vi "IVCV_measurement.vi"() -> ()   [LabVIEW 2016]
uses:
  <vilib>/Utility/file.llb/Read Delimited Spreadsheet (DBL).vi
panel:
  out "Channels":cluster{i32[], dbl[]}[](graph) caption="XY Graph"
  in  "Switch Delay (s)":dbl format="%#_13g"
  out "Voltages":cluster{"X":dbl[], "Y":dbl[]}[](graph) caption="XY Graph"
  in  "Voltage Delay (s)":dbl format="%#_13g"
  out "Input file":path
  in  "Sensor type":enum16{"6''", "8''"}(ring)
  in  "Measurement type":enum16{"IV", "CV"}(ring)
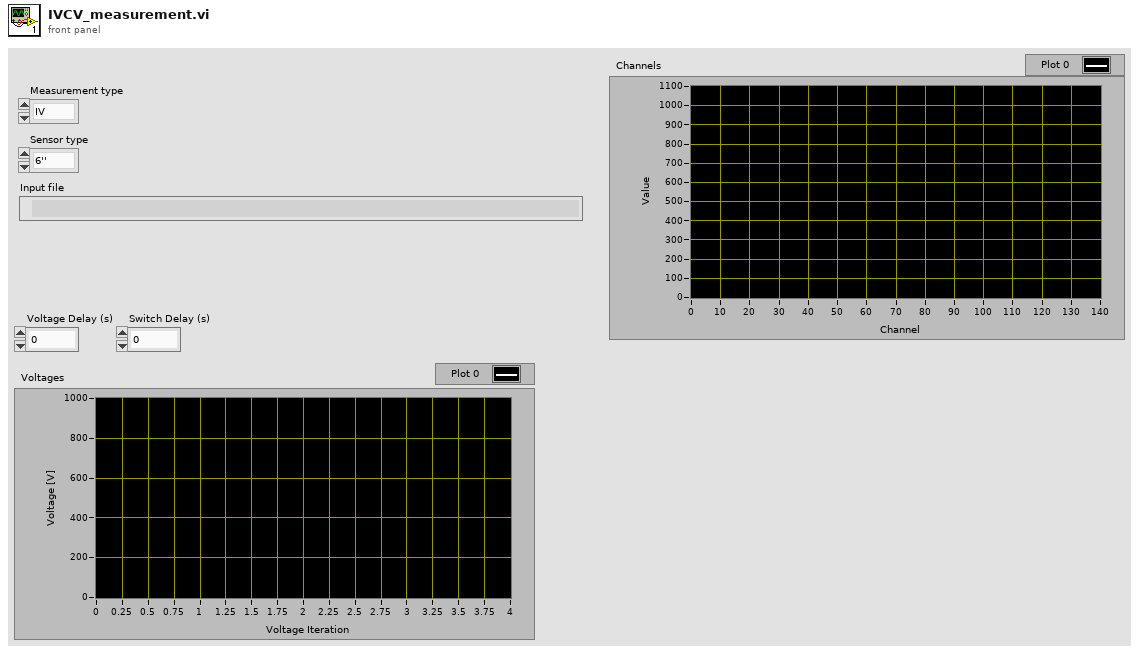
[diagram p1: front panel]
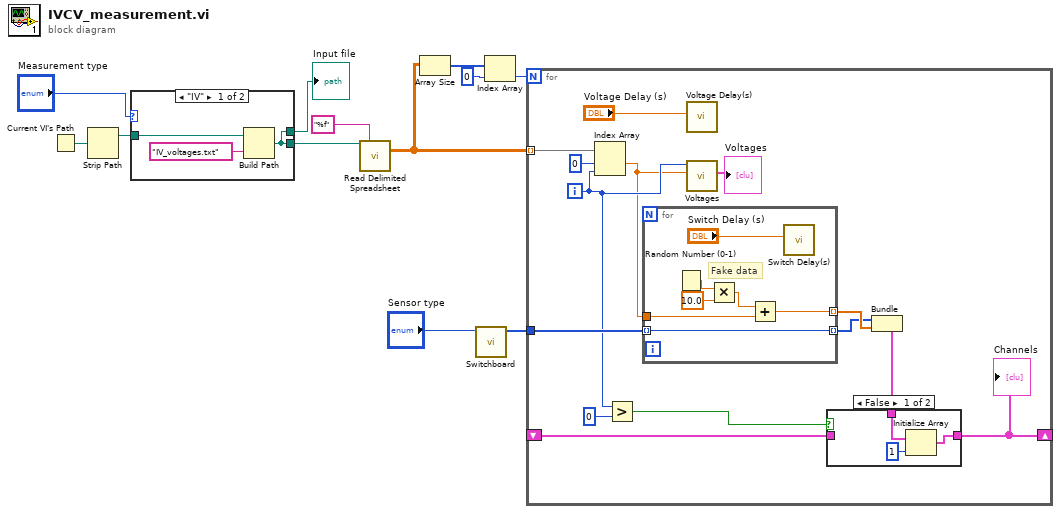
[diagram p0: block diagram]
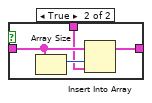
[diagram p2: hidden frame]
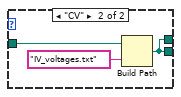
[diagram p3: hidden frame]
diagram:
  n1 = Current VI's Path() -> (path=w9:path)
  n2 = Strip Path(path=w9) -> (stripped path=w3:path)  [unwired: 1 out]
  n3 = case shown="\"IV\"" "Measurement type" {
    tunnel: [w13 w16] -> w11
    tunnel: w3 -> [w15 w17]
    tunnel: [w13 w16] -> w8
    frame "IV" {
      n4 = Build Path(base path=w15, name or relative path="IV_voltages.txt") -> (appended path=w13:path)
    }
    frame "CV" {
      n5 = Build Path(base path=w17, name or relative path="IV_voltages.txt") -> (appended path=w16:path)
    }
  }
  "Input file" <- w8
  n6 = call-poly <vilib>:"Read Delimited Spreadsheet.vi"("file path (dialog if empty)"=w11, "format (%.3f)"="%f") -> ("all rows"=w4:dbl[][])  [unwired: 8 in, 5 out]
  n7 = Array Size(array=w4) -> (size(s)=w7:i32[])
  n8 = call "Switchboard.vi"("Sensor type"="Sensor type") -> ("Output config"=w1:i32[])  [unwired: 10 in]
  n9 = Index Array(array=w7, index=0) -> (element=w5:i32)
  n10 = for {
    N: w5 -> [_]
    tunnel: w4 -> [w31] mode=indexing
    tunnel: w1 -> [w28]
    shift-right: [w24] -> _
    shift-left: _ -> [w27]
    i -> [w20]
    n11 = Index Array(array=w31, index #1=0 ("index"), index #2=w20) -> (element #1=w19:dbl)  [unwired: 1 out]
    n12 = Greater?(x=w20, y=0) -> (0:w21:bool)
    n13 = for {
      tunnel: w28 -> [w45] mode=indexing
      tunnel: [w45] -> w23 mode=indexing
      tunnel: [w41] -> w26 mode=indexing
      tunnel: w19 -> [w40]
      # "Fake data"
      n14 = Random Number (0-1)() -> (number: 0 to 1=w44:dbl)
      n15 = Multiply(x=w44, y=10.0) -> (x*y=w43:dbl)
      n16 = Add(x=w43, y=w40) -> (x+y=w41:dbl)
      n17 = call "Switch Delay(s)"("Delay Time (s)"="Switch Delay (s)") -> ()  [unwired: 10 in, 1 out]
    }
    n18 = call "Voltage Delay(s)"("Delay Time (s)"="Voltage Delay (s)") -> ()  [unwired: 10 in, 1 out]
    n19 = call "Voltages"("Y Input"=w19, "X Input"=w20) -> ("XY Graph"=→"Voltages":cluster{"X":dbl[], "Y":dbl[]}[])  [unwired: 8 in, 1 out]
    n20 = Bundle(w23, w26) -> (w25:cluster{i32[], dbl[]})  [unwired: 1 out]
    n21 = case shown="False" w21 {
      tunnel: w27 -> [_ w39]
      tunnel: w25 -> [w34 w37]
      tunnel: [w33 w36] -> w24
      frame False {
        n22 = Initialize Array(w34, 1 ("dimension size")) -> (w33:cluster{i32[], dbl[]}[])
      }
      frame True {
        n23 = Array Size(array=w39) -> (size(s)=w38:i32)
        n24 = Insert Into Array(array=w39, index=w38, new element=w37) -> (w36:cluster{i32[], dbl[]}[])
      }
    }
    "Channels" <- w24
  }
